vi "Rec Get Recordset Properties (R).vi"(4 "error in (no error)":errorcluster, 7 "recordset reference":T3) -> (0 "error out":errorcluster, 1 "recordset properties":T1, 3 "recordset reference out":T3)   [LabVIEW 2013, in "NI_Database_API_64.lvlib"]
doc: "Gets properties of the object as determined by the inputs. This VI works for connections, commands, recordsets, columns, and parameters. Wire data to the reference input to determine the polymorphic instance to use or manually select the instance."
uses:
  NI_Database_API_64.lvlib
  Rec ObjectReference.ctl
  Rec Properties.ctl
  Auxilliary.llb/DB Tools Cursor Type.ctl
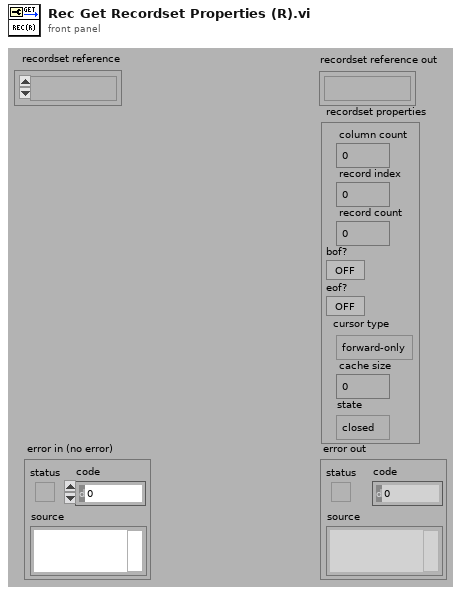
[diagram p1: front panel]
types:
  T1 = typedef "NI_Database_API_64.lvlib/Rec Properties.ctl" = cluster{"column count":i32, "record index":i32, "record count":i32, "bof?":bool, "eof?":bool, "cursor type":T2, "cache size":i32, "state":enum16{"closed", "open"}}
  T2 = typedef "NI_Database_API_64.lvlib/DB Tools Cursor Type.ctl" = enum16{"forward-only", "keyset", "dynamic", "static"}
  T3 = typedef "NI_Database_API_64.lvlib/Rec ObjectReference.ctl" = refnum<k1>
  T4 = typedef "NI_Database_API_64.lvlib/Rec DataMembers.ctl" = cluster{"ADODB._Recordset":refnum<k7>, "Connection":T5}
  T5 = typedef "NI_Database_API_64.lvlib/Conn ObjectReference.ctl" = refnum<k1>
  T6 = cluster{"Count":i32, "RecordCount":i32, "RecordCount":i32, "BOF":bool, "EOF":bool, "CursorType":i32, "CacheSize":i32, "State":i32}
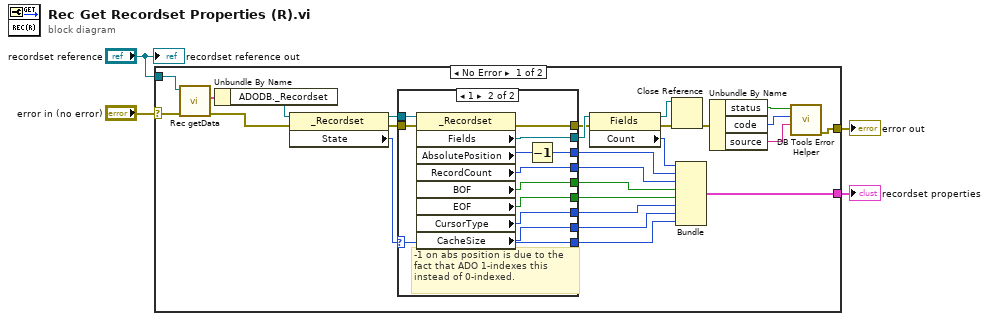
[diagram p0: block diagram]
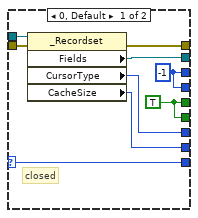
[diagram p2: hidden frame]
diagram:
  n1 = case shown="No Error" "error in (no error)" {
    selector: "error in (no error)" -> [w5 w52]
    tunnel: [w19 _] -> w4
    tunnel: "recordset reference" -> [w12 _]
    tunnel: [w7 w52] -> w3
    frame No Error {
      n2 = call "Rec getData.vi"("error in (no error)"=w5, "recordset reference"=w12) -> ("error out"=w11:errorcluster, "data"=w14:T4)  [unwired: 4 out]
      n3 = Unbundle By Name(w14) -> ("ADODB._Recordset"=w13:refnum<k7>)
      n4 = property class="_Recordset"(reference=w13, error in=w11) -> (reference out=w18:refnum<k7>, error out=w17:errorcluster, "State"=w16:i32)
      n5 = case shown="1" w16 {
        selector: w16 -> [w35 w43]
        tunnel: [w37 w51] -> w30
        tunnel: [w36 w50] -> w29
        tunnel: [w31 w42] -> w25
        tunnel: [w32 w49] -> w24
        tunnel: [w32 w48] -> w23
        tunnel: [w33 w47] -> w22
        tunnel: [w34 w46] -> w21
        tunnel: [w35 w43] -> w20
        tunnel: w18 -> [w38 w45]
        tunnel: w17 -> [w39 w44]
        tunnel: [w31 w40] -> w15
        frame 0, Default {
          w31 = -1 ("RecordCount")
          w32 = TRUE ("EOF")
          # "closed"
          n6 = property class="_Recordset"(reference=w38, error in=w39) -> (error out=w36:errorcluster, "Fields"=w37:refnum<k7>, "CursorType"=w33:i32, "CacheSize"=w34:i32)  [unwired: 1 out]
        }
        frame 1 {
          # "-1 on abs position is due to the \nfact that ADO 1-indexes this\ninstead of 0-indexed."
          n7 = property class="_Recordset"(reference=w45, error in=w44) -> (error out=w50:errorcluster, "Fields"=w51:refnum<k7>, "AbsolutePosition"=w41:i32, "RecordCount"=w42:i32, "BOF"=w49:bool, "EOF"=w48:bool, "CursorType"=w47:i32, "CacheSize"=w46:i32)  [unwired: 1 out]
          n8 = Decrement(x=w41) -> (x-1=w40:i32)
        }
      }
      n9 = property class="Fields"(reference=w30, error in=w29) -> (reference out=w26:refnum<k7>, error out=w27:errorcluster, "Count"=w28:i32)
      n10 = Close Reference(reference=w26, error in (no error)=w27) -> (error out=w8:errorcluster)
      n11 = Bundle("Count"=w28, "RecordCount"=w15, "RecordCount"=w25, "BOF"=w24, "EOF"=w23, "CursorType"=w22, "CacheSize"=w21, "State"=w20) -> (w19:T6)  [unwired: 1 out]
      n12 = Unbundle By Name(w8) -> ("status"=w9:bool, "code"=w6:i32, "source"=w10:string)
      n13 = call "DB Tools Error Helper.vi"("source"=w10, "code"=w6, "status"=w9) -> ("error out"=w7:errorcluster)  [unwired: 1 in, 7 out]
    }
    frame Error {
    }
  }
  "error out" <- w3
  "recordset properties" <- w4
  "recordset reference out" <- "recordset reference"
